vi "Dialog Get Team Number.vi"() -> (1 "Team Number":u32 caption="Password")   [LabVIEW 2025]
doc: "Displays a standard dialog box that prompts users to enter information, such as a user name and password.\n--------------------\n\nThis Express VI is configured as follows:\n\nMessage to Display to the User:Please enter the password\nThe inputs are: \nText Entry Box: Password"
uses:
  <vilib>/event_ctls.llb/eventvkey.ctl
panel:
  in  "Tab Control":enum32{"Page 1", "Page 2"}(tab)
  in  "Enter":bool
  in  "Team Number":string caption="Password"
  # "Enter Team Number"
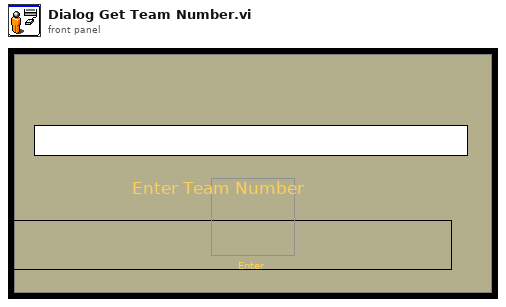
[diagram p1: front panel]
types:
  T1 = typedef "eventvkey.ctl" = enum16{"ASCII", "Enter", "Return", "Shift", "Ctrl", "Alt", "Cmd", "Opt", "Caps", "NumLock", "Clear", "Break", "Up", "Down", "Left", "Right", "Insert", "Delete", "Home", "End", "PageUp", "PageDown", "Escape", "Help", "Pause", "ScrollLock", "F1", "F2", "F3", "F4", "F5", "F6", "F7", "F8", "F9", "F10", "F11", "F12", "F13", "F14", "F15", "F16", "F17", "F18", "F19", "F20", "F21", "F22", "F23", "F24", "Play", "VolumeUp", "VolumeDown", "Mute", "Two Byte Char"}
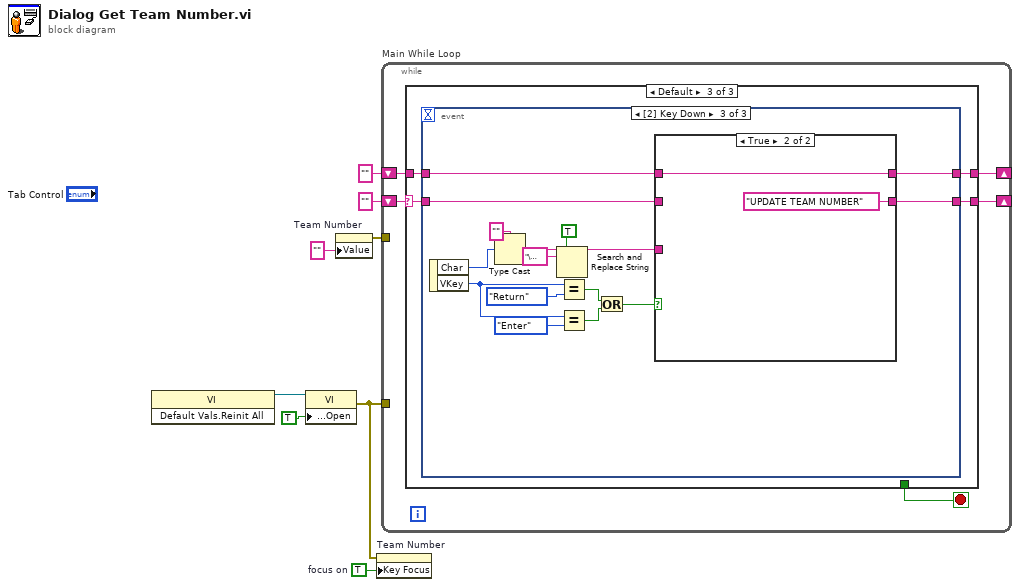
[diagram p0: block diagram]
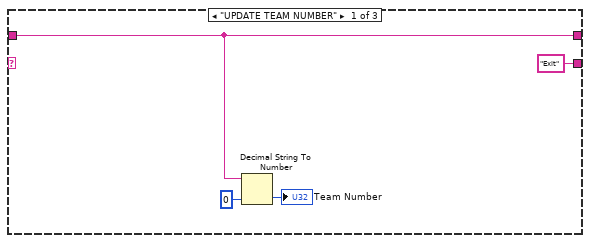
[diagram p2: hidden frame]
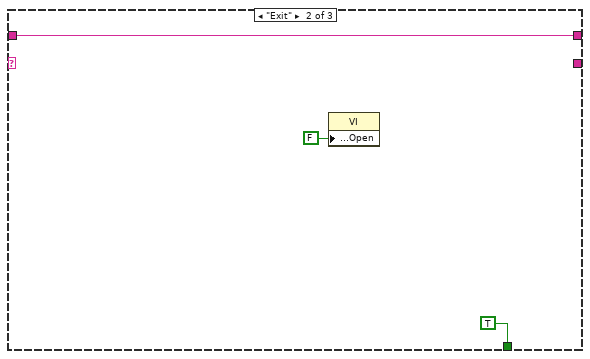
[diagram p3: hidden frame]
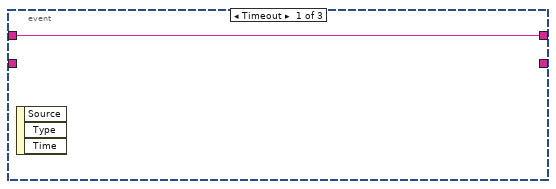
[diagram p4: hidden frame]
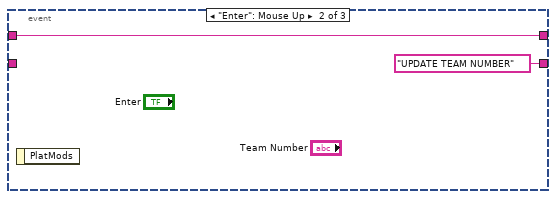
[diagram p5: hidden frame]
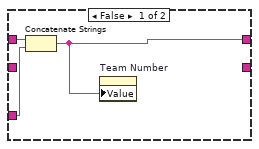
[diagram p6: hidden frame]
diagram:
  w6 = TRUE  # focus on
  n1 = invoke class="VI" method="Default Vals.Reinit All"() -> (reference out=w7:refnum<vi>)  [unwired: 3 in, 2 out]
  n2 = property class="VI"(reference=w7, "Front Panel Window:Open"=TRUE) -> (error out=w5:errorcluster)  [unwired: 1 in, 1 out]
  n3 = property on="Team Number" class="Str"("Value"="" ("Password in")) -> (error out=w1:errorcluster)  [unwired: 2 in, 1 out]
  n4 = property on="Team Number" class="Str"(error in=w5, "Key Focus"=w6) -> ()  [unwired: 1 in, 2 out]
  n5 = while "Main While Loop" {
    tunnel: w5 -> [_]
    shift-right: [w11] -> _
    shift-left: "" -> [w12]
    shift-right: [w9] -> _
    shift-left: "" -> [w10]
    tunnel: w1 -> [_]
    stop <- w13 stop-if-true
    n6 = case shown="Default" w12 {
      selector: w12 -> [_ _ w24]
      tunnel: [_ TRUE _] -> w13
      tunnel: ["Exit" _ w23] -> w11
      tunnel: w10 -> [w16 w19 w22]
      tunnel: [w16 w19 w21] -> w9
      frame "UPDATE TEAM NUMBER" {
        n7 = Decimal String To Number(string=w16, default (0L)=u32 0 ("default (0 I32)")) -> (number=→"Team Number":u32)  [unwired: 1 in, 1 out]
      }
      frame "Exit" {
        n8 = property class="VI"("Front Panel Window:Open"=FALSE) -> ()  [unwired: 2 in, 2 out]
      }
      frame Default {
        n9 = event shown="[2] Key Down" {
          selector: _ -> [_ _ _]
          dyn-events: _ -> [_ _ _]
          timeout: _ -> [_ _ _]
          tunnel: w24 -> [_ _ w37]
          tunnel: [_ "UPDATE TEAM NUMBER" w36] -> w23
          tunnel: w22 -> [w25 w26 w32]
          tunnel: [w25 w26 w33] -> w21
          event Timeout {
            n10 = event-data() -> ()  [unwired: 1 in, 3 out]
          }
          event "Enter": Mouse Up {
            n11 = event-data() -> ()  [unwired: 1 in, 1 out]
          }
          event Key Down {
            n12 = event-data() -> ("Char"=w35:i16, "VKey"=w41:T1)  [unwired: 1 in]
            n13 = Type Cast(type="", x=w35) -> (*(type *) &x=w31:string)
            n14 = Search and Replace String(replace all?=TRUE ("replace all? (F)"), input string=w31, search string="\u0000") -> (result string=w28:string)  [unwired: 5 in, 3 out]
            n15 = Equal?(x=w41, y=eventvkey."Return") -> (x = y?=w43:bool)
            n16 = Equal?(x=w41, y=eventvkey."Enter") -> (x = y?=w42:bool)
            n17 = Or(x=w43, y=w42) -> (x .or. y?=w38:bool)
            n18 = case shown="True" w38 {
              tunnel: w37 -> [_ _]
              tunnel: [_ "UPDATE TEAM NUMBER"] -> w36
              tunnel: w32 -> [w46 w47]
              tunnel: [w44 w47] -> w33
              tunnel: w28 -> [w45 _]
              frame False {
                n19 = Concatenate Strings(w46, w45) -> (w44:string)
                n20 = property on="Team Number" class="Str"("Value"=w44) -> ()  [unwired: 2 in, 2 out]
              }
              frame True {
              }
            }
          }
        }
      }
    }
  }
